vi "controlTest.vi"() -> ()   [LabVIEW 2014]
uses:
  <vilib>/event_ctls.llb/eventvkey.ctl
panel:
  in  "stop 2":bool
  out "Numeric 2":i32
  in  "stop":bool
  out "Numeric":i32
  out "VKey":T1
  out "Boolean":bool
  in  "Cancel Button":bool
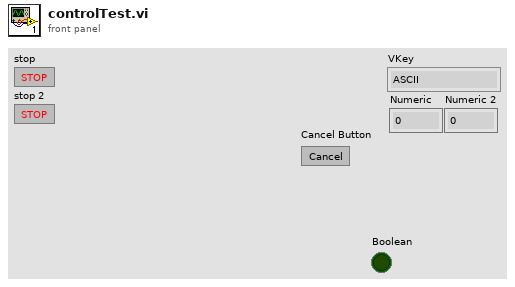
[diagram p1: front panel]
types:
  T1 = typedef "eventvkey.ctl" = enum16{"ASCII", "Enter", "Return", "Shift", "Ctrl", "Alt", "Cmd", "Opt", "Caps", "NumLock", "Clear", "Break", "Up", "Down", "Left", "Right", "Insert", "Delete", "Home", "End", "PageUp", "PageDown", "Escape", "Help", "Pause", "ScrollLock", "F1", "F2", "F3", "F4", "F5", "F6", "F7", "F8", "F9", "F10", "F11", "F12", "F13", "F14", "F15", "F16", "F17", "F18", "F19", "F20", "F21", "F22", "F23", "F24", "Play", "VolumeUp", "VolumeDown", "Mute", "Two Byte Char"}
  T2 = typedef "LVPositionTypeDef.ctl" = cluster{"Left":i32, "Top":i32}
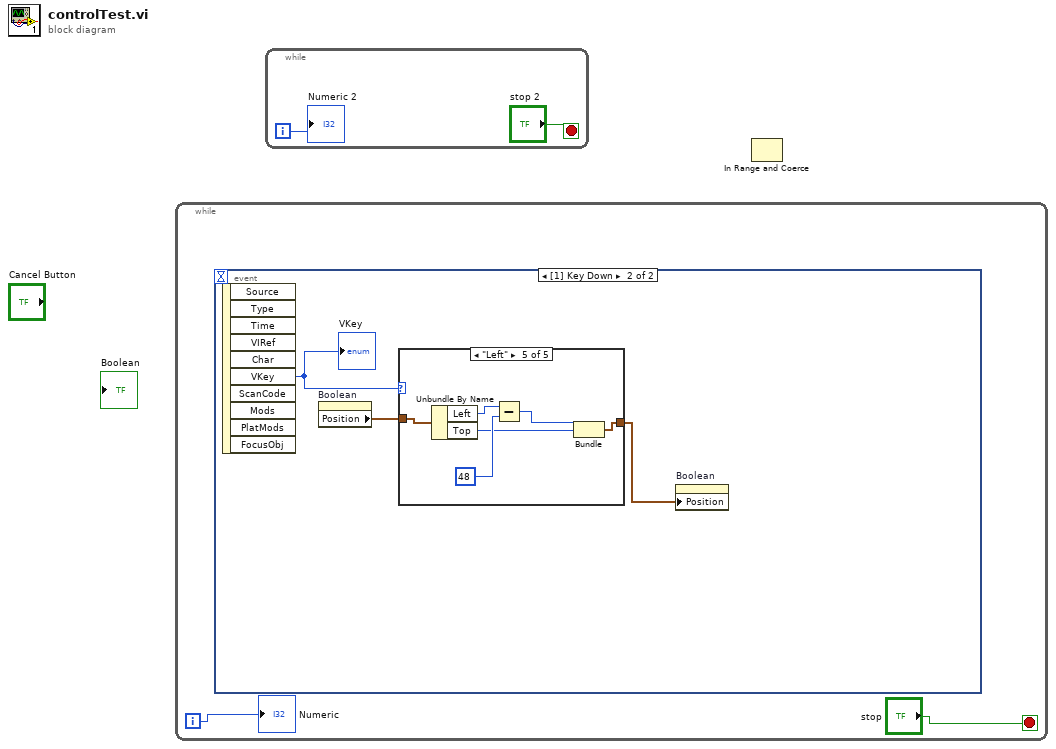
[diagram p0: block diagram]
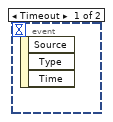
[diagram p2: hidden frame]
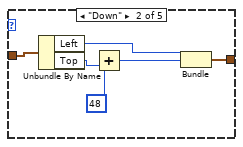
[diagram p4: hidden frame]
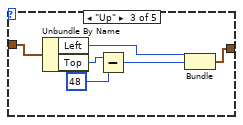
[diagram p5: hidden frame]
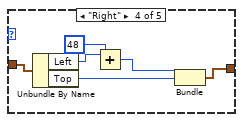
[diagram p6: hidden frame]
diagram:
  n1 = while {
    i -> [w2]
    stop <- "stop" stop-if-true
    n2 = event shown="[1] Key Down" {
      selector: _ -> [_ _]
      dyn-events: _ -> [_ _]
      timeout: _ -> [_ _]
      event Timeout {
        n3 = event-data() -> ()  [unwired: 1 in, 3 out]
      }
      event Key Down {
        n4 = event-data() -> ("VKey"=w5:T1)  [unwired: 1 in, 9 out]
        "VKey" <- w5
        n5 = property on="Boolean" class="Bool (strict)"() -> ("Position"=w4:T2)  [unwired: 2 in, 2 out]
        n6 = case shown="\"Left\"" w5 {
          tunnel: w4 -> [w6 w12 w16 w24 w26]
          tunnel: [w6 w8 w15 w19 w25] -> w3
          frame "ASCII", Default {
          }
          frame "Down" {
            n7 = Unbundle By Name(w12) -> ("Left"=w10:i32, "Top"=w11:i32)
            n8 = Add(x=48, y=w11) -> (x+y=w9:i32)
            n9 = Bundle("Left"=w10, w9) -> (w8:cluster{"Left":i32, i32})  [unwired: 1 in]
          }
          frame "Up" {
            n10 = Unbundle By Name(w16) -> ("Left"=w18:i32, "Top"=w14:i32)
            n11 = Subtract(x=w14, y=48) -> (x-y=w17:i32)
            n12 = Bundle("Left"=w18, w17) -> (w15:cluster{"Left":i32, i32})  [unwired: 1 in]
          }
          frame "Right" {
            n13 = Unbundle By Name(w24) -> ("Left"=w21:i32, "Top"=w23:i32)
            n14 = Add(x=w21, y=48) -> (x+y=w22:i32)
            n15 = Bundle(w22, "Top"=w23) -> (w19:cluster{i32, "Top":i32})  [unwired: 1 in]
          }
          frame "Left" {
            n16 = Unbundle By Name(w26) -> ("Left"=w29:i32, "Top"=w27:i32)
            n17 = Subtract(x=w29, y=48) -> (x-y=w28:i32)
            n18 = Bundle(w28, "Top"=w27) -> (w25:cluster{i32, "Top":i32})  [unwired: 1 in]
          }
        }
        n19 = property on="Boolean" class="Bool (strict)"("Position"=w3) -> ()  [unwired: 2 in, 2 out]
      }
    }
    "Numeric" <- w2
  }
  n20 = while {
    i -> [w32]
    stop <- "stop 2" stop-if-true
    "Numeric 2" <- w32
  }
  n21 = In Range and Coerce() -> ()  [unwired: 3 in, 2 out]
